vi "main.vi"() -> ()   [LabVIEW 2017]
panel:
  in  "CH4 Filename":path=path "test.tdms" caption="Filename"
  in  "LOX Filename":path=path "test.tdms" caption="Filename"
  out "CH4 Pressure":dynamicdata(graph)
  out "LOX Pressure":dynamicdata(graph)
  in  "CH4 Target Pressure (psi)":dbl
  in  "LOX Target Pressure (psi)":dbl
  in  "Regulate Pressure":bool
  in  "stop (F)":bool
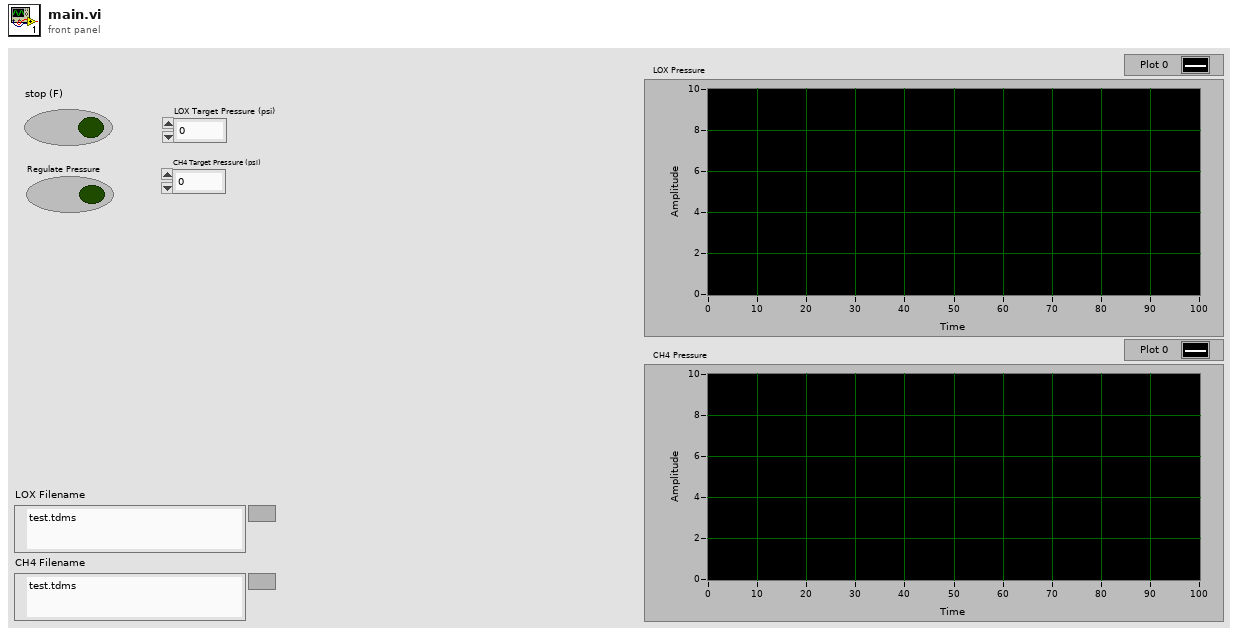
[diagram p1: front panel]
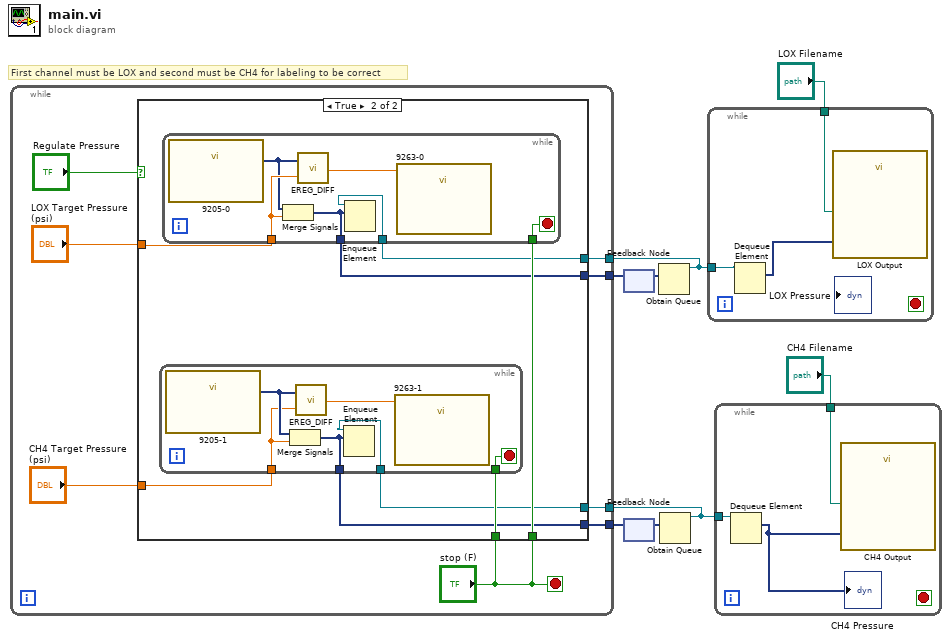
[diagram p0: block diagram]
diagram:
  # "First channel must be LOX and second must be CH4 for labeling to be correct"
  n1 = feedback #1() -> (w4:dynamicdata)  [unwired: 1 in]
  n2 = feedback #2() -> (w1:dynamicdata)  [unwired: 1 in]
  n3 = Obtain Queue(element data type=w4) -> (queue out=w6:refnum<queue>)  [unwired: 4 in, 2 out]
  n4 = Obtain Queue(element data type=w1) -> (queue out=w3:refnum<queue>)  [unwired: 4 in, 2 out]
  n5 = while {
    tunnel: w6 -> [w12]
    tunnel: [w11] -> w5
    tunnel: [w10] -> w2
    tunnel: w3 -> [w9]
    stop <- "stop (F)" stop-if-true
    n6 = case shown="True" "Regulate Pressure" {
      tunnel: "LOX Target Pressure (psi)" -> [_ w24]
      tunnel: "CH4 Target Pressure (psi)" -> [_ w23]
      tunnel: "stop (F)" -> [_ w22]
      tunnel: "stop (F)" -> [_ w21]
      tunnel: w12 -> [_ w20]
      tunnel: [_ w19] -> w11
      tunnel: [_ w18] -> w10
      tunnel: w9 -> [_ w17]
      frame False {
      }
      frame True {
        n7 = while {
          tunnel: w23 -> [w27]
          tunnel: w22 -> [w29]
          tunnel: [w26] -> w18
          tunnel: w17 -> [w25]
          stop <- w29 stop-if-true
          n8 = call "9205-1"() -> ("data"=w28:dynamicdata)  [unwired: 17 in, 2 out]
          n9 = Merge Signals(w28, w27) -> (w26:dynamicdata)
          n10 = call "EREG_DIFF.vi"("Target Pressure (psi)"=w27, "data"=w28) -> ("Output"=w30:dbl)
          n11 = Enqueue Element(queue=w25, element=w26) -> ()  [unwired: 2 in, 3 out]
          n12 = call "9263-1"("data"=w30) -> ()  [unwired: 17 in, 2 out]
        }
        n13 = while {
          tunnel: w24 -> [w34]
          tunnel: w21 -> [w35]
          tunnel: w20 -> [w31]
          tunnel: [w32] -> w19
          stop <- w35 stop-if-true
          n14 = call "9205-0"() -> ("data"=w33:dynamicdata)  [unwired: 17 in, 2 out]
          n15 = Merge Signals(w33, w34) -> (w32:dynamicdata)
          n16 = call "EREG_DIFF.vi"("Target Pressure (psi)"=w34, "data"=w33) -> ("Output"=w36:dbl)
          n17 = Enqueue Element(queue=w31, element=w32) -> ()  [unwired: 2 in, 3 out]
          n18 = call "9263-0"("data"=w36) -> ()  [unwired: 17 in, 2 out]
        }
      }
    }
  }
  n19 = feedback-in #1(w5) -> ()
  n20 = feedback-in #2(w2) -> ()
  n21 = while {
    tunnel: "LOX Filename" -> [w39]
    tunnel: w6 -> [w37]
    stop <- _ stop-if-true
    n22 = Dequeue Element(queue=w37) -> (element=w38:dynamicdata)  [unwired: 2 in, 3 out]
    n23 = call "LOX Output"("Signals"=w38, "Filename"=w39) -> ()  [unwired: 15 in, 3 out]
  }
  n24 = while {
    tunnel: "CH4 Filename" -> [w42]
    tunnel: w3 -> [w41]
    stop <- _ stop-if-true
    n25 = Dequeue Element(queue=w41) -> (element=w40:dynamicdata)  [unwired: 2 in, 3 out]
    "CH4 Pressure" <- w40
    n26 = call "CH4 Output"("Signals"=w40, "Filename"=w42) -> ()  [unwired: 15 in, 3 out]
  }
